vi "Remove invalid channels.vi"(8 "error in (no error)":errorcluster, 10 "engine configuration in":refnum<class "engine configuration.lvclass">, 11 "E2E configuration in":refnum<class "E2E Tag Exchange configuration.lvclass">) -> (0 "error out":errorcluster, 2 "engine configuration out":refnum<class "engine configuration.lvclass">, 3 "E2E configuration out":refnum<class "E2E Tag Exchange configuration.lvclass">)   [LabVIEW 2015, in "E2E Tag Exchange editor node.lvclass"]
uses:
  E2E Tag Exchange editor node.lvclass
  <vilib>/NI/Module Execution Interface/Engine Configuration/engine configuration.lvclass
  module/configuration/E2E Tag Exchange configuration.lvclass
  <vilib>/NI/Configuration Framework/serializable configuration/NISE_CEF_serializable configuration.lvclass/NISE_CEF_serializable configuration.ctl
  <vilib>/NI/Tag Bus/tag/tag descriptor.lvclass/tag descriptor.ctl
  <vilib>/Utility/LVClass/Get LV Class Name.vi
  <vilib>/NI/Configuration Framework/error generator/NISE_error generator.vi
  <vilib>/NI/Tag Bus/tag/tag descriptor.lvclass
  <vilib>/NI/Configuration Framework/serializable configuration/NISE_CEF_serializable configuration.lvclass
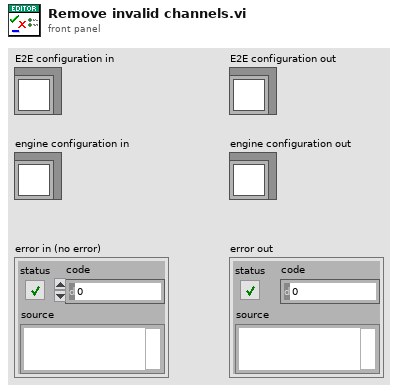
[diagram p1: front panel]
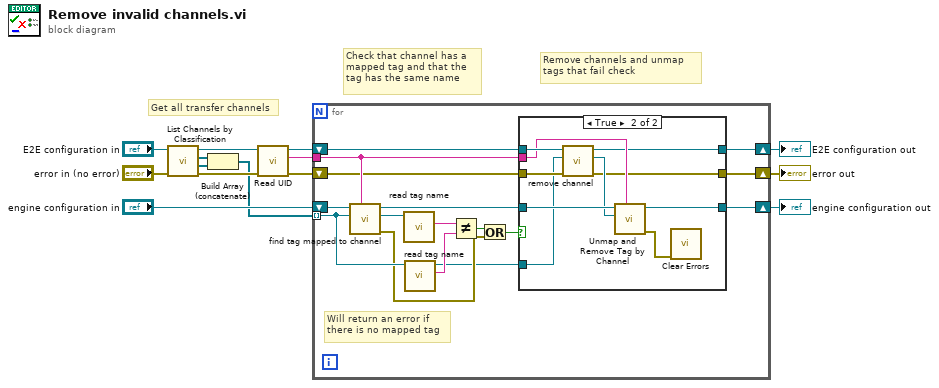
[diagram p0: block diagram]
diagram:
  # "Remove channels and unmap\ntags that fail check"
  # "Check that channel has a\nmapped tag and that the \ntag has the same name"
  # "Get all transfer channels"
  n1 = call "List Channels by Classification.vi"("E2E configuration in"="E2E configuration in") -> ("Output Channels"=w1:refnum<class "TBM channel.lvclass">[], "Input Channels"=w8:refnum<class "TBM channel.lvclass">[], "E2E configuration out"=w9:refnum<class "E2E Tag Exchange configuration.lvclass">)  [unwired: 8 in]
  n2 = Build Array (concatenate)(w8, w1) -> (w2:refnum<class "TBM channel.lvclass">[])
  n3 = call <vilib>:"Read UID.vi"("error in"="error in (no error)", "configuration in"=w9) -> ("error out"=w13:errorcluster, "instance id"=w11:string, "configuration out"=w10:refnum<class "E2E Tag Exchange configuration.lvclass">)  [unwired: 7 in]
  n4 = for {
    tunnel: w2 -> [w28] mode=indexing
    tunnel: w11 -> [w22]
    shift-right: [w14] -> w5
    shift-left: w10 -> [w24]
    shift-right: [w21] -> w3
    shift-left: "engine configuration in" -> [w29]
    shift-right: [w15] -> w4
    shift-left: w13 -> [w17]
    # "Will return an error if\nthere is no mapped tag"
    n5 = call <vilib>:"find tag mapped to channel.vi"("owner"=w22, "channel"=w28, "engine configuration in"=w29) -> ("error out"=w18:errorcluster, "tag"=w27:refnum<class "tag descriptor.lvclass">, "engine configuration out"=w23:refnum<class "engine configuration.lvclass">)  [unwired: 6 in]
    n6 = call <vilib>:"read tag name.vi"("system tag in"=w27) -> ("name"=w26:string)  [unwired: 8 in, 2 out]
    n7 = call <vilib>:"read tag name.vi"("system tag in"=w28) -> ("name"=w25:string, "system tag out"=w16:refnum<class "TBM channel.lvclass">)  [unwired: 8 in, 1 out]
    n8 = Not Equal?(x=w26, y=w25) -> (x != y?=w20:bool)
    n9 = Or(x=w20, y=w18) -> (x .or. y?=w19:bool)
    n10 = case shown="True" w19 {
      tunnel: w24 -> [w32 w42]
      tunnel: w23 -> [w30 w41]
      tunnel: w22 -> [_ w35]
      tunnel: [w30 w38] -> w21
      tunnel: w17 -> [w31 w37]
      tunnel: w16 -> [_ w36]
      tunnel: [w31 w34] -> w15
      tunnel: [w32 w33] -> w14
      frame False {
      }
      frame True {
        n11 = call "remove channel.vi"("error in (no error)"=w37, "channel"=w36, "E2E configuration in"=w42) -> ("error out"=w34:errorcluster, "removed channel"=w40:refnum<class "TBM channel.lvclass">, "E2E configuration out"=w33:refnum<class "E2E Tag Exchange configuration.lvclass">)  [unwired: 6 in]
        n12 = call "Unmap and Remove Tag by Channel.vi"("owner ID"=w35, "channel"=w40, "engine configuration in"=w41) -> ("error out"=w39:errorcluster, "engine configuration out"=w38:refnum<class "engine configuration.lvclass">)  [unwired: 7 in]
        n13 = call <vilib>:"Clear Errors.vi"("error in (no error)"=w39) -> ()  [unwired: 5 in, 2 out]
      }
    }
  }
  "E2E configuration out" <- w5
  "error out" <- w4
  "engine configuration out" <- w3
